vi "Add ClientID Session.vi"(8 "error in (no error)":errorcluster, 9 "SessionMailbox":refnum<queue>, 10 "Client ID":string, 11 "MQTT_Base in":refnum<class "MQTT_Base.lvclass">) -> (0 "error out":errorcluster, 3 "MQTT_Base out":refnum<class "MQTT_Base.lvclass">)   [LabVIEW 2013, in "MQTT Server.lvlib" / "MQTT_Base.lvclass"]
uses:
  MQTT_Base.lvclass
  Response -- cluster.ctl
  Control Packets/ControlPacket/ControlPacket.lvclass
  SessionRef -- cluster.ctl
  MQTT_Base.lvclass/MQTT_Base.ctl
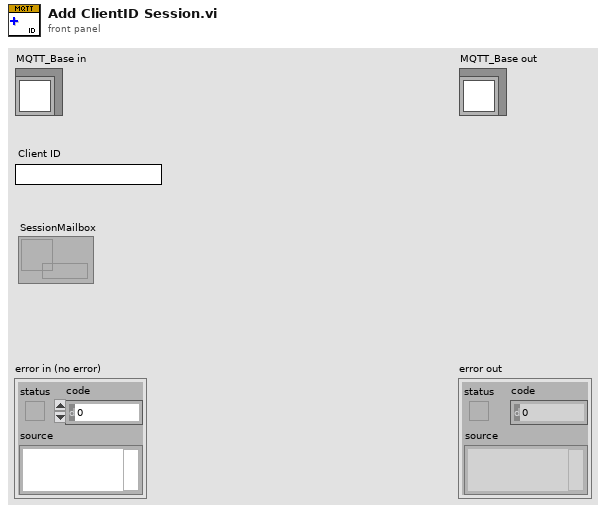
[diagram p1: front panel]
types:
  T1 = typedef "MQTT Server.lvlib/MQTT_Base.lvclass/SessionRef -- cluster.ctl" = cluster{"ClientID":string, "SessionMailbox":refnum<queue>}
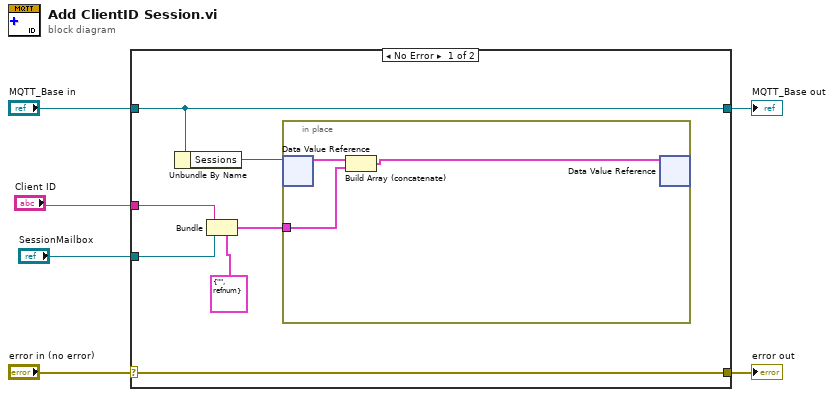
[diagram p0: block diagram]
diagram:
  n1 = case shown="No Error" "error in (no error)" {
    selector: "error in (no error)" -> [w8 w18]
    tunnel: [w8 w18] -> w5
    tunnel: [w13 w17] -> w3
    tunnel: "MQTT_Base in" -> [w13 w17]
    tunnel: "Client ID" -> [w11 _]
    tunnel: "SessionMailbox" -> [w10 _]
    frame No Error {
      n2 = Unbundle By Name(w13) -> ("Sessions"=w12:refnum<data-value>)
      n3 = Bundle(cluster=T1 {"ClientID"="", "SessionMailbox"=refnum} ("SessionRef"), "ClientID"=w11, "SessionMailbox"=w10) -> (w7:T1)
      n4 = in-place {
        in-place-border: w7 -> [w15]
        n5 = in-place-dvr #1(w12) -> (w16:T1[])  [unwired: 1 out]
        n6 = Build Array (concatenate)(w16, w15) -> (w14:T1[])
        n7 = in-place-dvr #1(w14) -> ()  [unwired: 2 out]
      }
    }
    frame Error {
    }
  }
  "error out" <- w5
  "MQTT_Base out" <- w3
